vi "Build.vi"(8 "error in (no error)":errorcluster, 10 "Send Builder in":refnum<class "Send Builder.lvclass">, 11 "Message Maker in":refnum<class "Message Scripter.lvclass">) -> (0 "error out":errorcluster, 2 "Send Builder out":refnum<class "Send Builder.lvclass">, 3 "Message Maker out":refnum<class "Message Scripter.lvclass">)   [LabVIEW 2020, in "Message Maker.lvlib" / "Send Builder.lvclass"]
uses:
  Send Builder.lvclass
  Message Scripter/Message Scripter.lvclass
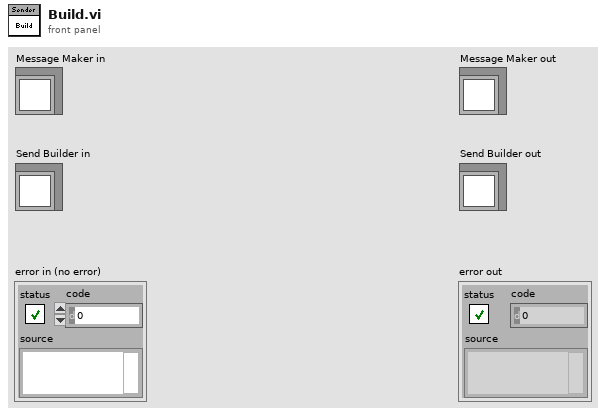
[diagram p1: front panel]
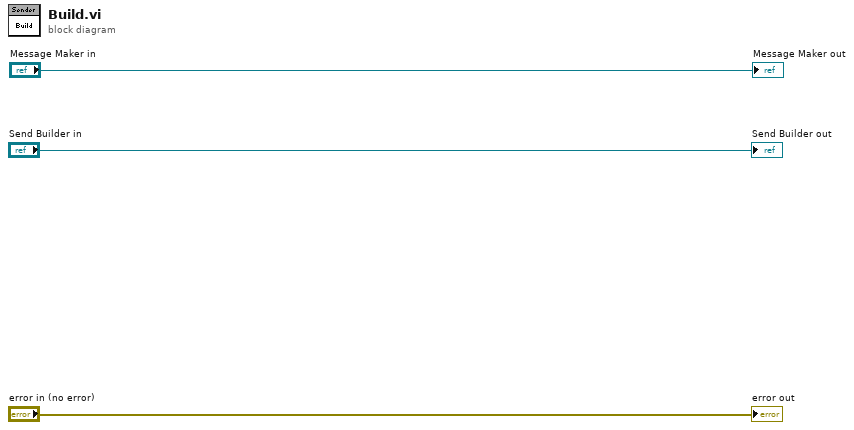
[diagram p0: block diagram]
diagram:
  "error out" <- "error in (no error)"
  "Send Builder out" <- "Send Builder in"
  "Message Maker out" <- "Message Maker in"
